vi "rsscope Read Waveform.vi"(0 "VISA resource name":refnum<visa-resource-name>, 1 "Waveform (1)":i32=1, 5 "Channel (1)":i32(ring)=1 items=["1"=1, "2"=2, "3"=3, "4"=4], 9 "Maximum Time (5000)":i32=5000, 11 "error in (no error)":errorcluster) -> (4 "VISA resource name out":refnum<visa-resource-name>, 6 "Waveform Array":dbl[](array[numeric]) format="%^.3e", 10 "Initial X":dbl format="%^.3e", 14 "X Increment":dbl format="%^.3e", 15 "error out":errorcluster)   [LabVIEW 2018]
doc: "This VI initiates an acquisition on the channels that you enable with the rsscope Configure Channel.vi. It then waits for the acquisition to complete, and returns the waveform for the channel you specify. You call the rsscope Fetch Waveform.vi to obtain the waveforms for each of the remaining enabled channels without initiating another acquisition.\n\nNotes:\n- After this VI executes, each element in the Waveform Array parameter is either a voltage or a value indicating that the oscilloscope could not sample a voltage.\n- You configure the interpolation method the oscilloscope uses with the rsscope Configure Interpolation.vi. If you disable interpolation, the oscilloscope does not interpolate points in the waveform.\n\nAttribute:\n-\n\nRemote-control commands:\nSINGle\n*OPC\nCHANnel<m>[:WAVeform<n>]:DATA[:VALues]"
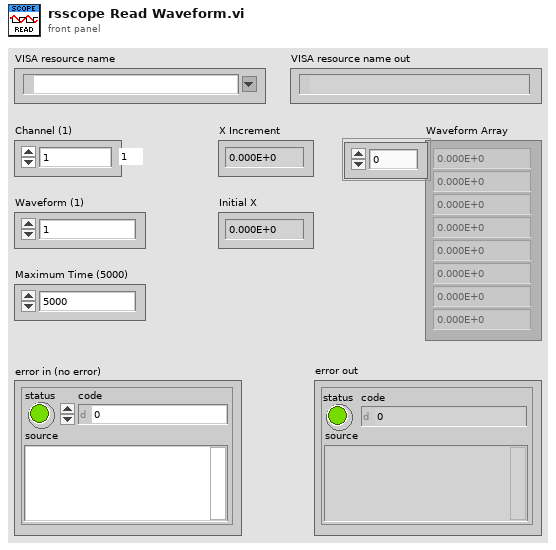
[diagram p1: front panel]
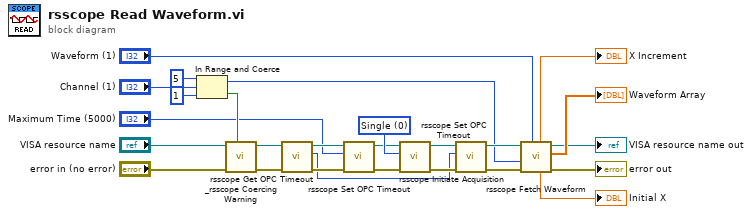
[diagram p0: block diagram]
diagram:
  w16 = 0 items=["Single", "Continuous", "Force"] ("Action (Single)")
  n1 = In Range and Coerce(upper limit=5, x="Channel (1)", lower limit=1) -> (coerced(x)=w2:i32, In Range?=w21:bool)
  n2 = call "_rsscope Coercing Warning.vi"("In Range?"=w21, "error in (no error)"="error in (no error)", "VISA resource name"="VISA resource name") -> ("error out"=w14:errorcluster, "VISA resource name out"=w15:refnum<visa-resource-name>)  [unwired: 7 in]
  n3 = call "rsscope Get OPC Timeout.vi"("error in (no error)"=w14, "VISA resource name"=w15) -> ("error out"=w6:errorcluster, "OPC Timeout"=w1:i32, "VISA resource name out"=w7:refnum<visa-resource-name>)  [unwired: 7 in]
  n4 = call "rsscope Set OPC Timeout.vi"("error in (no error)"=w6, "OPC Timeout (15000)"="Maximum Time (5000)", "VISA resource name"=w7) -> ("error out"=w8:errorcluster, "VISA resource name out"=w9:refnum<visa-resource-name>)  [unwired: 7 in]
  n5 = call "rsscope Initiate Acquisition.vi"("error in (no error)"=w8, "Action (Single)"=w16, "VISA resource name"=w9) -> ("error out"=w12:errorcluster, "VISA resource name out"=w13:refnum<visa-resource-name>)  [unwired: 7 in]
  n6 = call "rsscope Set OPC Timeout.vi"("error in (no error)"=w12, "OPC Timeout (15000)"=w1, "VISA resource name"=w13) -> ("error out"=w10:errorcluster, "VISA resource name out"=w11:refnum<visa-resource-name>)  [unwired: 7 in]
  n7 = call "rsscope Fetch Waveform.vi"("Waveform (1)"="Waveform (1)", "error in (no error)"=w10, "Channel (1)"=w2, "VISA resource name"=w11) -> ("error out"=→"error out":errorcluster, "Waveform Array"=→"Waveform Array":dbl[], "VISA resource name out"=→"VISA resource name out":refnum<visa-resource-name>, "Initial X"=→"Initial X":dbl, "X Increment"=→"X Increment":dbl)  [unwired: 3 in]
